vi "Query Registry.vi"(8 "error in":errorcluster, 11 "Name In":string) -> (0 "error out":errorcluster, 1 "Found":bool, 2 "Alias":string, 3 "Name Out":string)   [LabVIEW 2019, in "Identifier.lvclass"]
uses:
  Identifier.lvclass
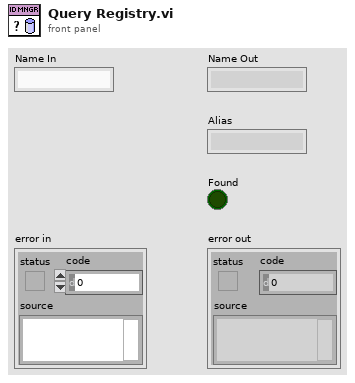
[diagram p1: front panel]
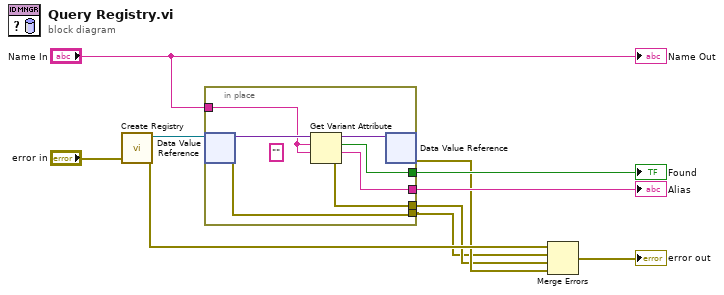
[diagram p0: block diagram]
diagram:
  n1 = call "Create Registry.vi"("error in"="error in") -> ("error out"=w5:errorcluster, "Registry"=w9:refnum<data-value>)  [unwired: 9 in]
  n2 = in-place {
    in-place-border: "Name In" -> [w11]
    in-place-border: [w16] -> w7
    in-place-border: [w14] -> w6
    in-place-border: [w13] -> w1
    in-place-border: [w12] -> w2
    (unwired) ""
    n3 = in-place-dvr #1(w9) -> (w17:variant, w13:errorcluster)
    n4 = Get Variant Attribute(Variant=w17, name=w11, default value (empty Variant)=w11) -> (duplicate Variant=w15:variant, found=w14:bool, value=w16:string, error out=w12:errorcluster)  [unwired: 1 in]
    n5 = in-place-dvr #1(w15) -> (w3:errorcluster)  [unwired: 1 out]
  }
  "Alias" <- w7
  "Found" <- w6
  n6 = Merge Errors(w5, w1, w2, w3) -> (→"error out":errorcluster)
  "Name Out" <- "Name In"
